vi "Handle Drag Starting.vi"(4 "Mods":cluster{"Double Click":bool, "Menu Key":bool}, 5 "Drag Mode":enum32{"copy or move", "copy only", "move only"}(ring), 6 "PlatMods":T3, 7 "Button":u16, 8 "error in (no error)":errorcluster, 9 "Coords":T2, 10 "Data":T4(array[cluster]), 11 "Test Executive View in":refnum<class "Test Executive View.lvclass">) -> (0 "error out":errorcluster, 2 "Drag Starting Filtered Event Data":T1, 3 "Test Executive View out":refnum<class "Test Executive View.lvclass">)   [LabVIEW 2019, in "Test Executive View.lvclass"]
uses:
  <vilib>/gpm_packages/@cs/Test-executive-builder/Example/Application/Test Executive View/Test Executive View/Test Executive View.lvclass
  C:/Program Files/National Instruments/LabVIEW 2019/vi.lib/gpm_packages/@cs/Test-executive-builder/Source/Test Executive Builder View/Test Executive Builder View/Test Executive Builder View.lvclass
  <vilib>/Utility/miscctls.llb/LVPoint32TypeDef.ctl
  <vilib>/gpm_packages/@cs/Test-executive-builder/Source/Application Dependencies/Drag Starting Filtered Event Data.ctl
  <vilib>/gpm_packages/@cs/Test-executive-builder/Source/Test Executive Builder View/Test Executive Builder View/Test Executive Builder View.lvclass/Test Executive Builder View.ctl
  <vilib>/gpm_packages/@cs/Test-executive-builder/Source/Test Executive Builder View/Tree Click Interpreter/Tree Click Interpreter.lvclass
  <vilib>/gpm_packages/@cs/Test-executive-builder/Source/Test Executive Builder View/Test Executive Builder View/Test Executive Builder View.lvclass
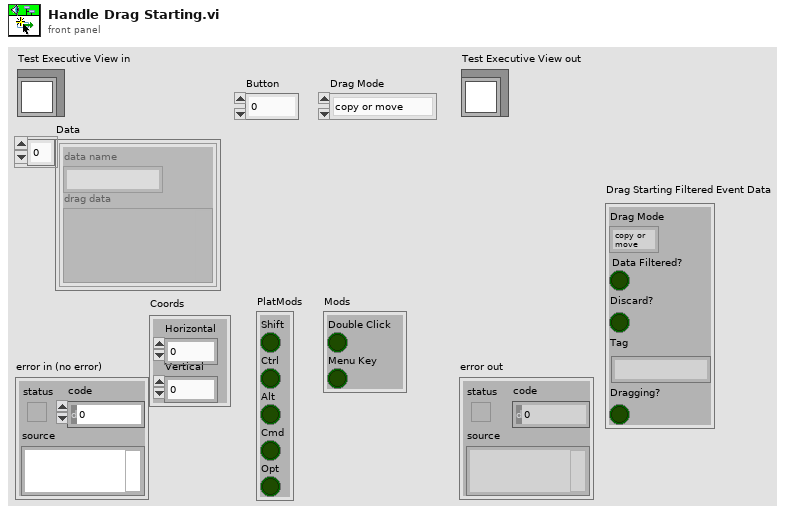
[diagram p1: front panel]
types:
  T1 = typedef "Drag Starting Filtered Event Data.ctl" = cluster{"Drag Mode":enum32{"copy or move", "copy only", "move only"}, "Data Filtered?":bool, "Discard?":bool, "Tag":string, "Dragging?":bool}
  T2 = typedef "LVPoint32TypeDef.ctl" = cluster{"Horizontal":i32, "Vertical":i32}
  T3 = cluster{"Shift":bool, "Ctrl":bool, "Alt":bool, "Cmd":bool, "Opt":bool}
  T4 = cluster{"data name":string, "drag data":variant}[]
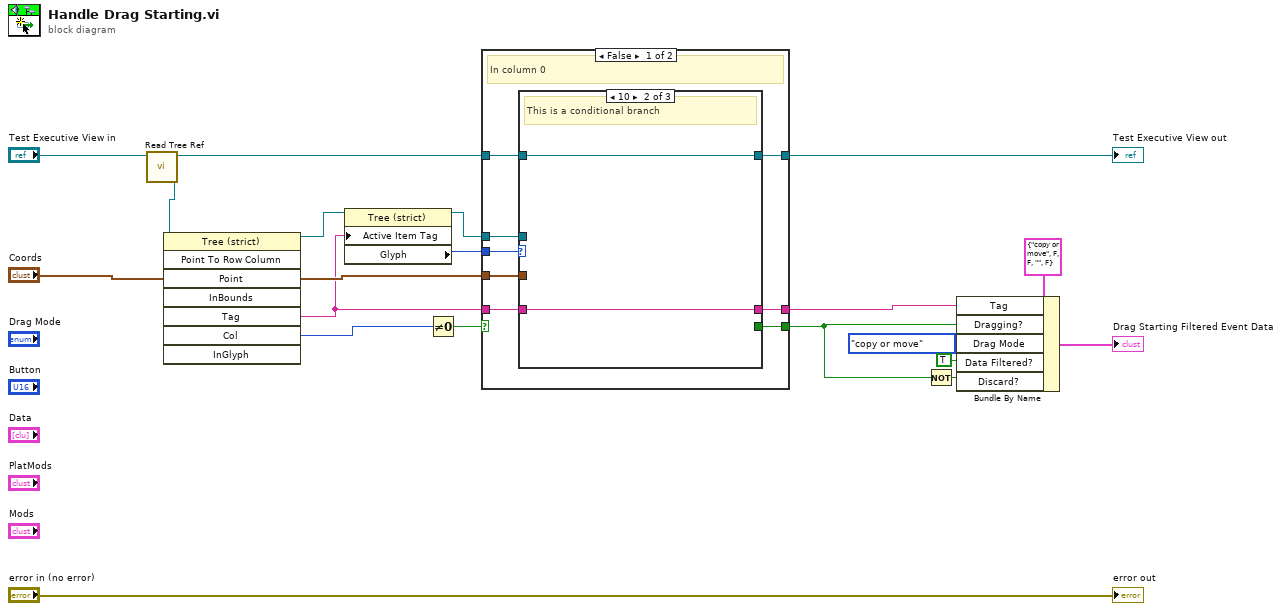
[diagram p0: block diagram]
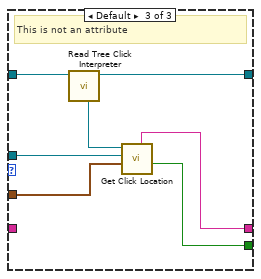
[diagram p3: hidden frame]
diagram:
  n1 = call <vilib>:"Read Tree Ref.vi"("Test Executive Builder View in"="Test Executive View in") -> ("Tree Ref"=w16:refnum<vi>, "Test Executive Builder View out"=w9:refnum<class "Test Executive View.lvclass">)  [unwired: 9 in]
  n2 = invoke class="Tree (strict)" method="Point To Row Column"(reference=w16, "Point"="Coords") -> (reference out=w4:refnum<vi>, "Tag"=w2:string, "Col"=w15:i32)  [unwired: 6 in, 5 out]
  n3 = property class="Tree (strict)"(reference=w4, "Active Item Tag"=w2) -> (reference out=w3:refnum<vi>, "Glyph"=w1:i32)  [unwired: 1 in, 1 out]
  n4 = Not Equal To 0?(x=w15) -> (x != 0?=w14:bool)
  n5 = case shown="False" w14 {
    selector: w14 -> [_ w41]
    tunnel: w2 -> [w20 w40]
    tunnel: "Coords" -> [w24 _]
    tunnel: w3 -> [w25 _]
    tunnel: [w22 w41] -> w5
    tunnel: [w23 w40] -> w6
    tunnel: [w26 w39] -> w8
    tunnel: w9 -> [w27 w39]
    tunnel: w1 -> [w21 _]
    frame False {
      # "In column 0"
      n6 = case shown="10" w21 {
        tunnel: w27 -> [w29 w31 w38]
        tunnel: [w29 w31 w37] -> w26
        tunnel: w25 -> [_ _ w35]
        tunnel: w24 -> [_ _ w34]
        tunnel: [w28 w30 w33] -> w23
        tunnel: [_ _ w32] -> w22
        tunnel: w20 -> [w28 w30 _]
        frame 5 {
          # "This is an attribute"
        }
        frame 10 {
          # "This is a conditional branch"
        }
        frame Default {
          # "This is not an attribute"
          n7 = call <vilib>:"Read Tree Click Interpreter.vi"("Test Executive Builder View in"=w38) -> ("Test Executive Builder View out"=w37:refnum<class "Test Executive View.lvclass">, "Tree Click Interpreter"=w36:refnum<class "Tree Click Interpreter.lvclass">)  [unwired: 9 in]
          n8 = call-dynamic "Get Click Location.vi"("Coords"=w34, "Tree Refnum"=w35, "Tree Click Interpreter in"=w36) -> ("Valid?"=w32:bool, "Tag"=w33:string)  [unwired: 4 in, 3 out]
        }
      }
    }
    frame True {
      # "Not in column 0"
    }
  }
  "Test Executive View out" <- w8
  n9 = Not(x=w5) -> (.not. x?=w7:bool)
  n10 = Bundle By Name(cluster=T1 {"Drag Mode"=enum."copy or move", "Data Filtered?"=FALSE, "Discard?"=FALSE, "Tag"="", "Dragging?"=FALSE} ("Drag Starting Filtered Event Data"), "Tag"=w6, "Dragging?"=w5, "Drag Mode"=enum32{"copy or move", "copy only", "move only"}."copy or move", "Data Filtered?"=TRUE, "Discard?"=w7) -> (→"Drag Starting Filtered Event Data":T1)
  "error out" <- "error in (no error)"
